vi "Create.vi"(8 "error in (no error)":errorcluster) -> (0 "error out":errorcluster, 3 "GW-PickUp-Cmd out":refnum<class "GW-PickUp-Cmd.lvclass">)   [LabVIEW 2013, in "GW-PickUp-Cmd.lvclass"]
uses:
  GW-PickUp-Cmd.lvclass
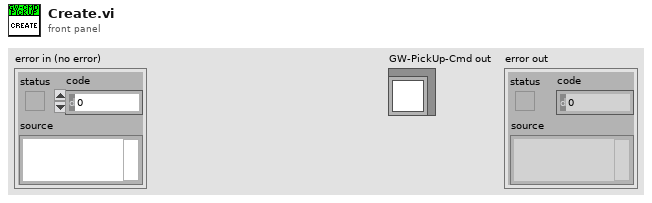
[diagram p1: front panel]
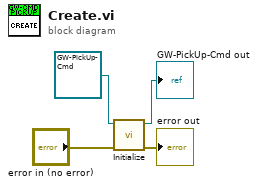
[diagram p0: block diagram]
diagram:
  n1 = call-dynamic "Initialize.vi"("error in (no error)"="error in (no error)", "GW-PickUp-Cmd in"=refnum<class "GW-PickUp-Cmd.lvclass"> refnum ("GW-PickUp-Cmd.lvclass")) -> ("error out"=→"error out":errorcluster, "GW-PickUp-Cmd out"=→"GW-PickUp-Cmd out":refnum<class "GW-PickUp-Cmd.lvclass">)  [unwired: 8 in]
